vi "ManualMode.vi"(8 "error in (no error)":errorcluster, 10 "MainUI":refnum<queue>, 11 "ManualModeQueue":refnum<queue>) -> (0 "error out":errorcluster)   [LabVIEW 2019, in "ManualMode.lvlib"]
uses:
  ManualMode.lvlib
  Cluster - ManualModeMessageCluster.ctl
  Enum - ManualModeMessage.ctl
  MainController/Cluster - MainControllerMessage.ctl
  MainController/Enum - MainState.ctl
  Cluster - ManualModeData.ctl
  MainController/Cluster - HardwareConfiguration.ctl
  Cluster - ManualModeMonitorMessage.ctl
  Enum - ManualModeMonitorState.ctl
  Cluster - UIRefs.ctl
  Mark10 API/WriteSpeed.vi
  Mark10 API/WriteCWTravelLimit.vi
  Mark10 API/WriteCCWTravelLimit.vi
  Mark10 API/WriteStopMove.vi
  Mark10 API/WriteResetPositionToZero.vi
  MainController/MainController.lvlib
  Mark10 API/Mark 10 TSTM-DC.lvlib
  Utilites/Utilities.lvlib
panel:
  out "Work":dbl format="%.2f"
  out "Torque":dbl format="%.2f N"
  out "Position":dbl format="%.2f °"
  in  "GotoZero":bool
  in  "StopMove":bool
  in  "MoveCW":bool
  in  "MoveCCW":bool
  in  "SetZero":bool
  in  "Speed":dbl format="%.2f °/s"
  in  "Angle":dbl format="%.2f °"
  in  "CommandBar":cluster{"Start":bool, "Stop":bool}
  out "Wf":waveform(dbl)[](graph)
  in  "Pause":bool
  # "Mark 10 Control"
  # "Moves CW to 0"
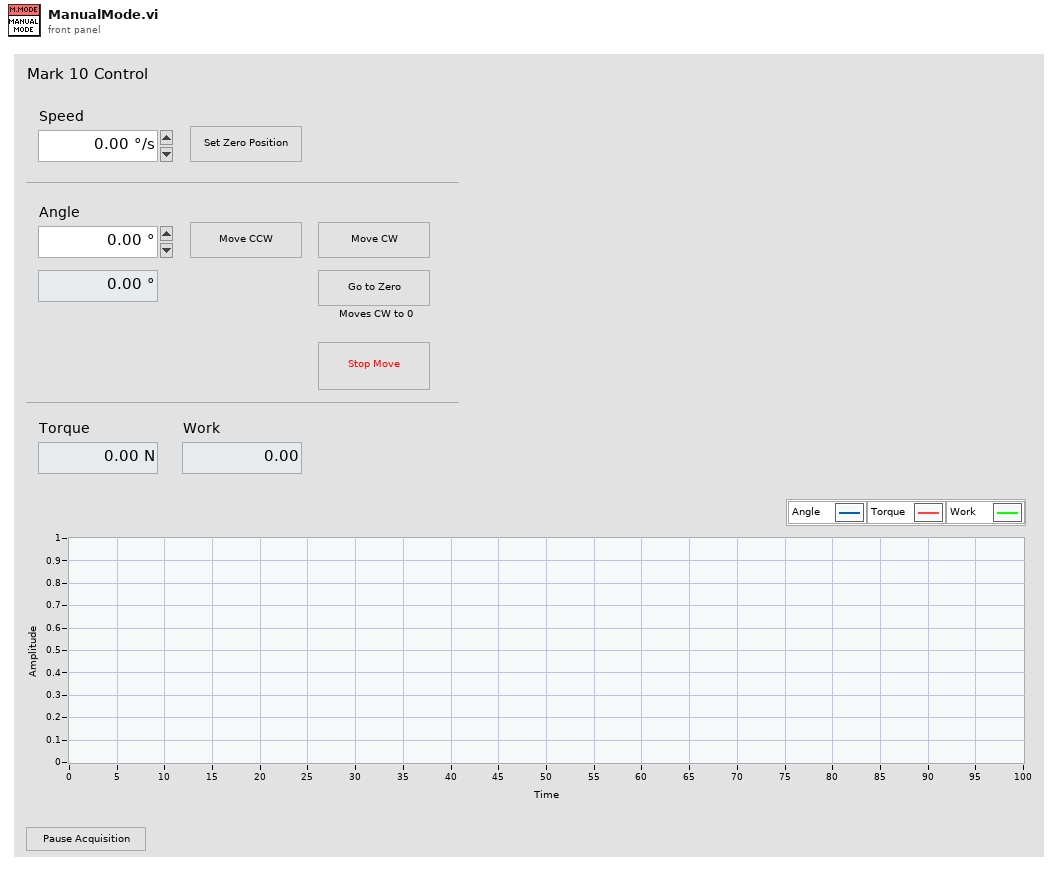
[diagram p1: front panel]
types:
  T1 = typedef "ManualMode.lvlib/Enum - ManualModeMonitorState.ctl" = enum16{"Idle", "SetCOM", "SetUIRefs", "Start", "Read", "Stop", "Pause", "Exit"}
  T2 = typedef "ManualMode.lvlib/Cluster - ManualModeMonitorMessage.ctl" = cluster{"Message":T1, "Data":variant}
  T3 = typedef "ManualMode.lvlib/Cluster - ManualModeData.ctl" = cluster{"Hardware Configuration":T4, "UIRefs":cluster{"Speed":refnum<vi>, "Angle":refnum<vi>}}
  T4 = typedef "MainController.lvlib/Cluster - HardwareConfiguration.ctl" = cluster{"Mark10COM":refnum<visa-resource-name>, "IsConnected":bool}
  T5 = typedef "ManualMode.lvlib/Enum - ManualModeMessage.ctl" = enum16{"Initialize", "Idle", "Start", "Stop", "Pause", "Resume", "BroadcastPreCollection", "MoveCCW", "MoveCW", "StopMove", "SetZero", "GotoZero", "UpdateHW", "Error", "Exit"}
  T6 = typedef "ManualMode.lvlib/Cluster - UIRefs.ctl" = cluster{"Work":refnum<vi>, "Torque":refnum<vi>, "Position":refnum<vi>, "Wf":refnum<vi>}
  T7 = typedef "MainController.lvlib/Enum - MainState.ctl" = enum16{"Initialize", "InitUIRefs", "LaunchSettings", "LaunchAutoMode", "LaunchManualMode", "LaunchTestReport", "ConnectHardware", "DisconnectHardware", "HiliteNavItems", "StartAutoMode", "PauseAutoMode", "StopAutoMode", "ShowFlyout", "HideFlyout", "BroadcastSettings", "PickupTestSettings", "BroadcastHW", "AutoTestDone", "DAQStatus", "UpdateCommandBar", "Error", "RecieveError", "Exit"}
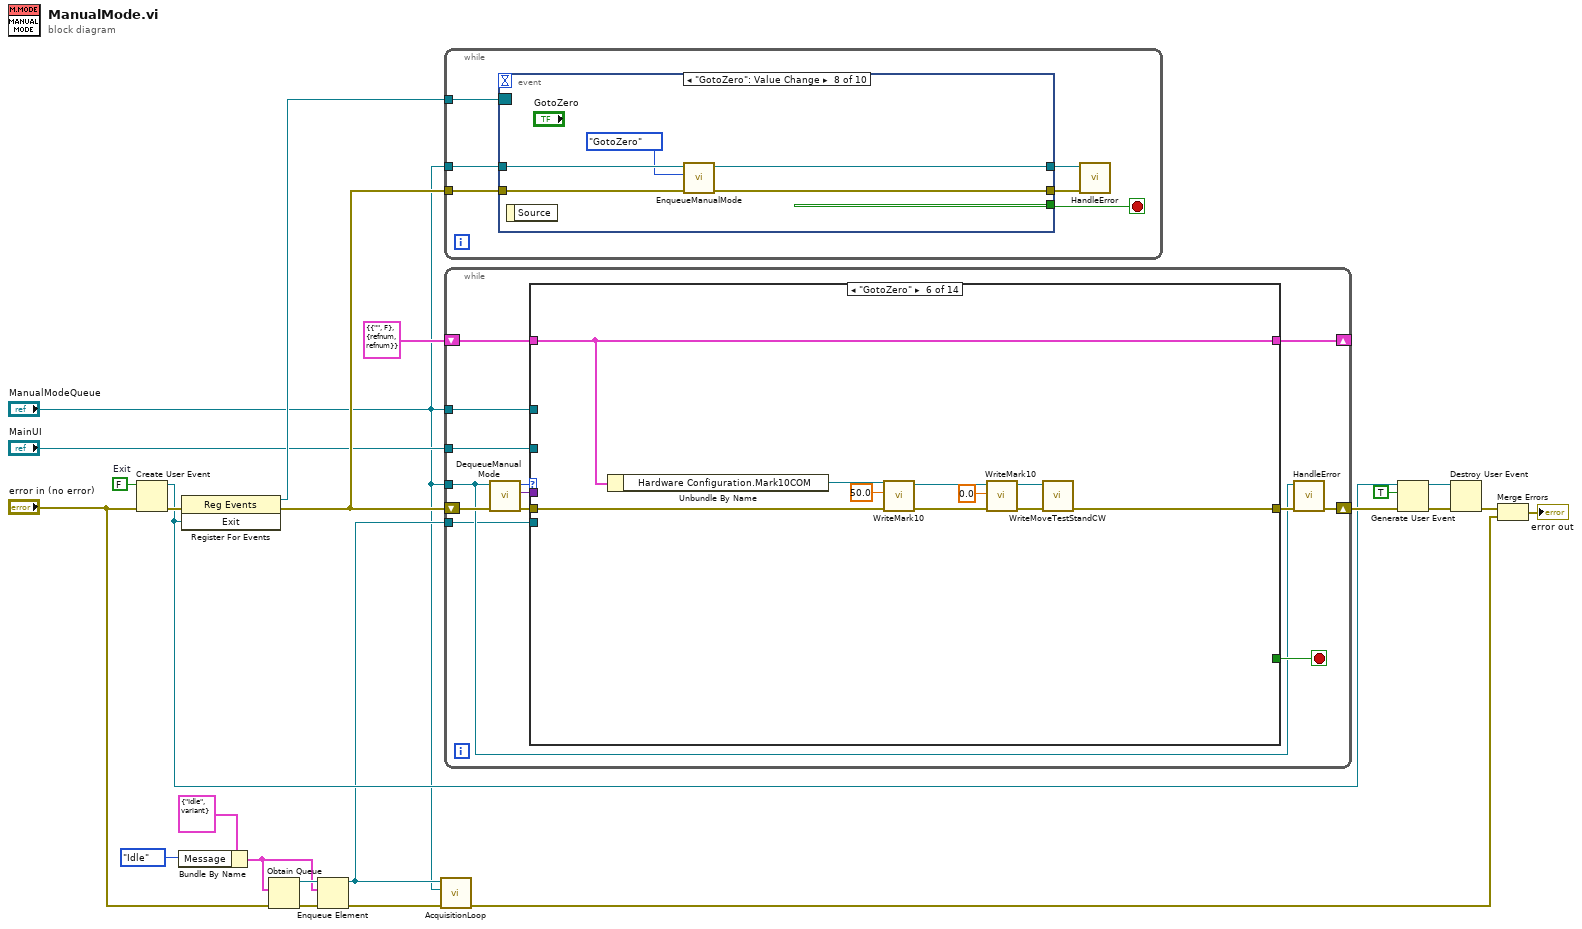
[diagram p0: block diagram]
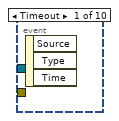
[diagram p2: hidden frame]
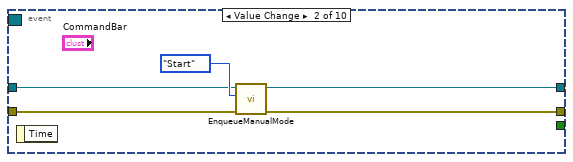
[diagram p3: hidden frame]
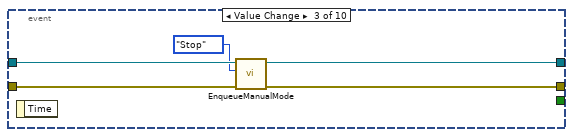
[diagram p4: hidden frame]
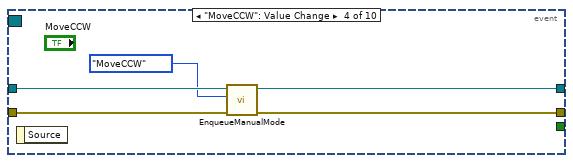
[diagram p5: hidden frame]
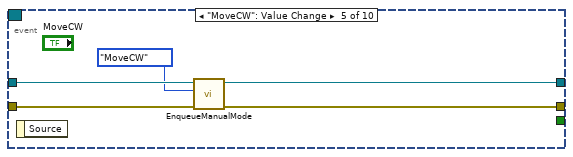
[diagram p6: hidden frame]
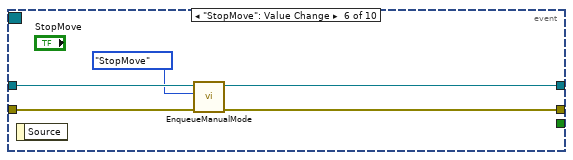
[diagram p7: hidden frame]
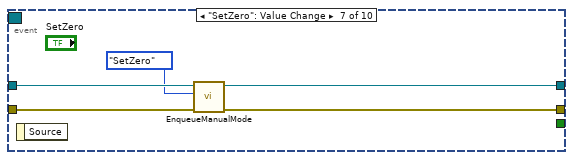
[diagram p8: hidden frame]
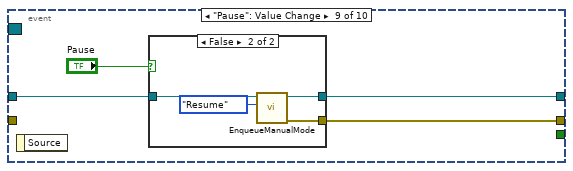
[diagram p9: hidden frame]
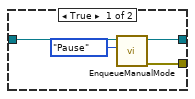
[diagram p10: hidden frame]
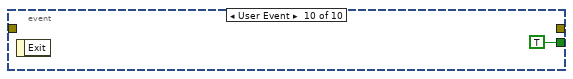
[diagram p11: hidden frame]
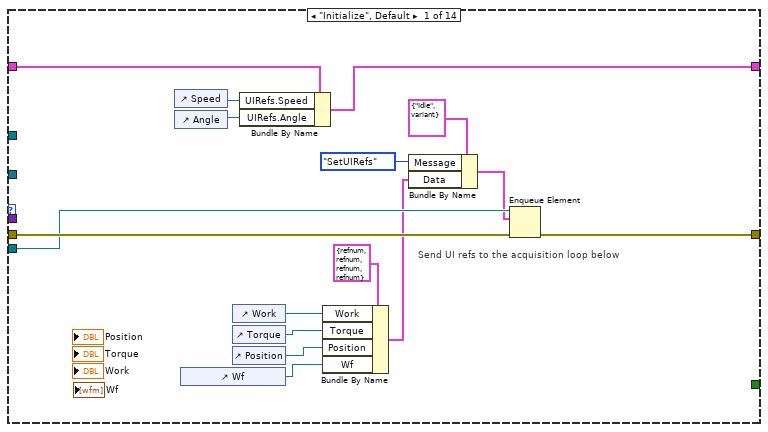
[diagram p12: hidden frame]
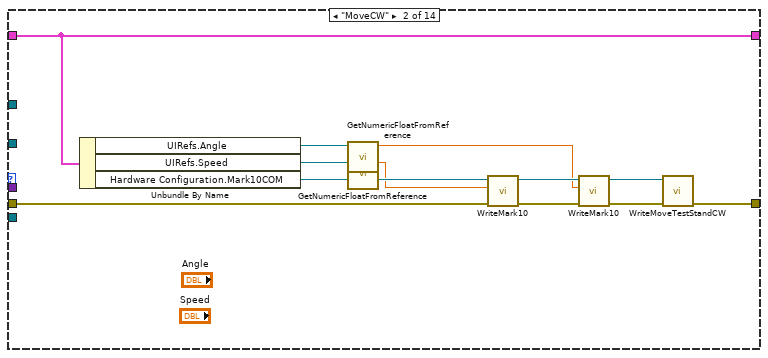
[diagram p13: hidden frame]
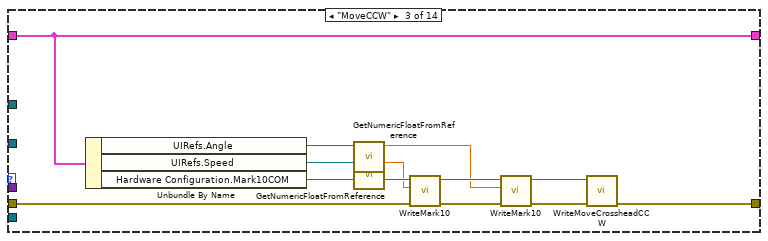
[diagram p14: hidden frame]
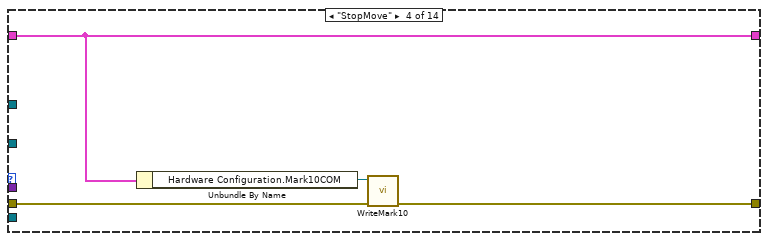
[diagram p15: hidden frame]
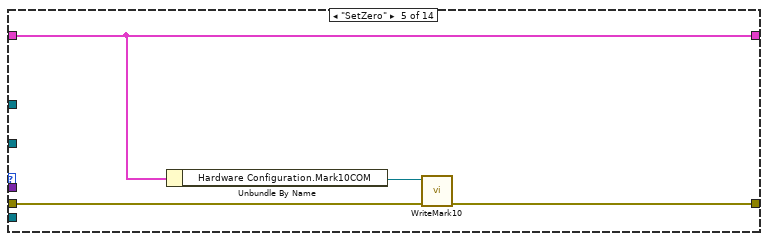
[diagram p16: hidden frame]
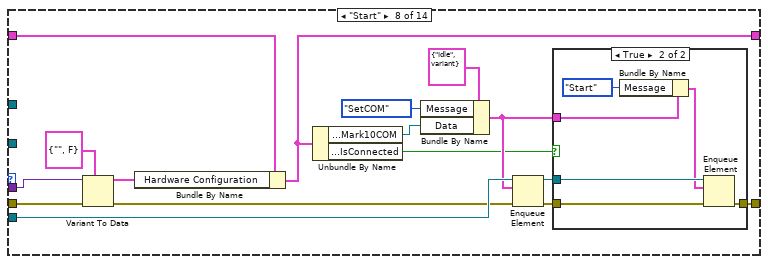
[diagram p18: hidden frame]
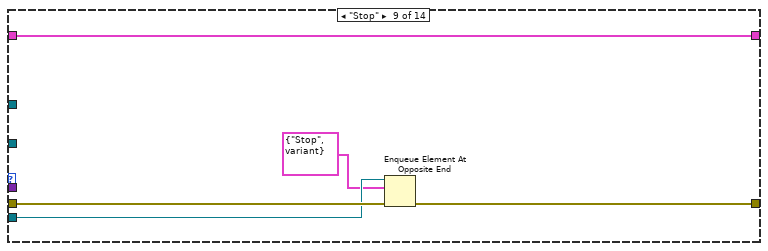
[diagram p20: hidden frame]
diagram:
  w22 = FALSE  # Exit
  n1 = Create User Event(user event datatype=w22, error in="error in (no error)") -> (user event=w19:refnum<user-event>, error out=w23:errorcluster)
  n2 = Bundle By Name(cluster=T2 {"Message"=enum."Idle", "Data"=variant}, "Message"=Enum_-_ManualModeMonitorState."Idle") -> (w6:T2)
  n3 = register-events(error in=w23, w19) -> (reference out=w21:refnum<event-registration>, error out=w14:errorcluster)  [unwired: 1 in]
  n4 = Obtain Queue(element data type=w6, error in (no error)="error in (no error)") -> (queue out=w10:refnum<queue>, error out=w11:errorcluster)  [unwired: 3 in, 1 out]
  n5 = Enqueue Element(queue=w10, element=w6, error in (no error)=w11) -> (queue out=w5:refnum<queue>, error out=w9:errorcluster)  [unwired: 1 in, 1 out]
  n6 = call "AcquisitionLoop.vi"("error in (no error)"=w9, "ManualModeQueue"="ManualModeQueue", "AcquisitionQueue"=w5) -> ("Error Out"=w3:errorcluster)  [unwired: 8 in]
  n7 = while {
    tunnel: w21 -> [w29]
    tunnel: w14 -> [w27]
    tunnel: "ManualModeQueue" -> [w26]
    stop <- w28 stop-if-true
    n8 = event shown="[7] \"GotoZero\": Value Change" {
      selector: w29 -> [_ _ _ _ _ _ _ _ _ _]
      dyn-events: _ -> [_ _ _ _ _ _ _ _ _ _]
      timeout: _ -> [_ _ _ _ _ _ _ _ _ _]
      tunnel: [_ _ _ _ _ _ _ _ _ TRUE] -> w28
      tunnel: w27 -> [_ w34 w39 w43 w48 w53 w58 w63 _ _]
      tunnel: w26 -> [_ w32 w38 w44 w49 w54 w59 w64 w68 _]
      tunnel: [_ w30 w35 w40 w45 w50 w55 w60 w67 _] -> w25
      tunnel: [_ w31 w36 w41 w46 w51 w56 w61 w66 _] -> w24
      event Timeout {
        n9 = event-data() -> ()  [unwired: 1 in, 3 out]
      }
      event "CommandBar.Start": Value Change {
        n10 = event-data() -> ()  [unwired: 1 in, 1 out]
        n11 = call "EnqueueManualMode.vi"("error in (no error)"=w34, "Message"=Enum_-_ManualModeMessage."Start" ("PreCollectionMessage"), "queue"=w32) -> ("error out"=w30:errorcluster, "queue out"=w31:refnum<queue>)  [unwired: 7 in]
      }
      event "CommandBar.Stop": Value Change {
        n12 = event-data() -> ()  [unwired: 1 in, 1 out]
        n13 = call "EnqueueManualMode.vi"("error in (no error)"=w39, "Message"=Enum_-_ManualModeMessage."Stop" ("PreCollectionMessage"), "queue"=w38) -> ("error out"=w35:errorcluster, "queue out"=w36:refnum<queue>)  [unwired: 7 in]
      }
      event "MoveCCW": Value Change {
        n14 = event-data() -> ()  [unwired: 1 in, 1 out]
        n15 = call "EnqueueManualMode.vi"("error in (no error)"=w43, "Message"=Enum_-_ManualModeMessage."MoveCCW", "queue"=w44) -> ("error out"=w40:errorcluster, "queue out"=w41:refnum<queue>)  [unwired: 7 in]
      }
      event "MoveCW": Value Change {
        n16 = event-data() -> ()  [unwired: 1 in, 1 out]
        n17 = call "EnqueueManualMode.vi"("error in (no error)"=w48, "Message"=Enum_-_ManualModeMessage."MoveCW", "queue"=w49) -> ("error out"=w45:errorcluster, "queue out"=w46:refnum<queue>)  [unwired: 7 in]
      }
      event "StopMove": Value Change {
        n18 = event-data() -> ()  [unwired: 1 in, 1 out]
        n19 = call "EnqueueManualMode.vi"("error in (no error)"=w53, "Message"=Enum_-_ManualModeMessage."StopMove", "queue"=w54) -> ("error out"=w50:errorcluster, "queue out"=w51:refnum<queue>)  [unwired: 7 in]
      }
      event "SetZero": Value Change {
        n20 = event-data() -> ()  [unwired: 1 in, 1 out]
        n21 = call "EnqueueManualMode.vi"("error in (no error)"=w58, "Message"=Enum_-_ManualModeMessage."SetZero", "queue"=w59) -> ("error out"=w55:errorcluster, "queue out"=w56:refnum<queue>)  [unwired: 7 in]
      }
      event "GotoZero": Value Change {
        n22 = event-data() -> ()  [unwired: 1 in, 1 out]
        n23 = call "EnqueueManualMode.vi"("error in (no error)"=w63, "Message"=Enum_-_ManualModeMessage."GotoZero", "queue"=w64) -> ("error out"=w60:errorcluster, "queue out"=w61:refnum<queue>)  [unwired: 7 in]
      }
      event "Pause": Value Change {
        n24 = event-data() -> ()  [unwired: 1 in, 1 out]
        n25 = case shown="False" "Pause" {
          tunnel: w68 -> [w72 w76]
          tunnel: [w70 w74] -> w67
          tunnel: [w69 w73] -> w66
          frame True {
            n26 = call "EnqueueManualMode.vi"("Message"=Enum_-_ManualModeMessage."Pause", "queue"=w72) -> ("error out"=w70:errorcluster, "queue out"=w69:refnum<queue>)  [unwired: 8 in]
          }
          frame False {
            n27 = call "EnqueueManualMode.vi"("Message"=Enum_-_ManualModeMessage."Resume", "queue"=w76) -> ("error out"=w74:errorcluster, "queue out"=w73:refnum<queue>)  [unwired: 8 in]
          }
        }
      }
      event User Event {
        n28 = event-data() -> ()  [unwired: 1 in, 1 out]
      }
    }
    n29 = call "HandleError.vi"("error in (no error)"=w25, "queue"=w24) -> ()  [unwired: 8 in, 2 out]
  }
  n30 = while {
    tunnel: "ManualModeQueue" -> [w79]
    shift-right: [w80] -> w20
    shift-left: w14 -> [w90]
    shift-right: [w85] -> _
    shift-left: T3 {"Hardware Configuration"={"Mark10COM"="", "IsConnected"=FALSE}, "UIRefs"={"Speed"=refnum, "Angle"=refnum}} -> [w86]
    tunnel: "MainUI" -> [w83]
    tunnel: "ManualModeQueue" -> [w82]
    tunnel: w5 -> [w78]
    stop <- w87 stop-if-true
    n31 = call "DequeueManualMode.vi"("error in (no error)"=w90, "Queue in"=w79) -> ("error out"=w88:errorcluster, "Data"=w89:variant, "State"=w84:T5)  [unwired: 7 in]
    n32 = case shown="\"GotoZero\"" w84 {
      tunnel: w89 -> [_ _ _ _ _ _ _ w158 _ _ _ w198 w203 _]
      tunnel: [w105 w112 w126 w133 w137 w140 w150 w162 w176 w181 w186 w194 w207 w212] -> w81
      tunnel: w88 -> [w106 w116 w130 w134 w138 w145 w150 w166 w177 w183 w188 w200 w202 _]
      tunnel: [_ _ _ _ _ _ _ _ _ _ _ _ _ TRUE] -> w87
      tunnel: w86 -> [w93 w118 w122 w132 w136 w147 w149 w153 w178 w182 w187 w195 w208 w213]
      tunnel: [w94 w118 w122 w132 w136 w147 w149 w154 w178 w182 w187 w196 w208 w213] -> w85
      tunnel: w83 -> [_ _ _ _ _ _ _ _ _ _ _ _ w206 _]
      tunnel: w82 -> [_ _ _ _ _ _ _ _ _ _ _ _ _ _]
      tunnel: w78 -> [w104 _ _ _ _ _ _ w165 w175 w180 w185 w193 _ w211]
      frame "Initialize", Default {
        # "Send UI refs to the acquisition loop below"
        n33 = control-ref of="Speed"() -> (w92:refnum<vi>)
        n34 = control-ref of="Angle"() -> (w91:refnum<vi>)
        n35 = control-ref of="Wf"() -> (w103:refnum<vi>)
        n36 = control-ref of="Work"() -> (w100:refnum<vi>)
        n37 = control-ref of="Torque"() -> (w101:refnum<vi>)
        n38 = control-ref of="Position"() -> (w102:refnum<vi>)
        n39 = Bundle By Name(cluster=w93, "UIRefs.Speed"=w92, "UIRefs.Angle"=w91) -> (w94:T3)
        n40 = Bundle By Name(cluster=T6 {"Work"=refnum, "Torque"=refnum, "Position"=refnum, "Wf"=refnum} ("output cluster"), "Work"=w100, "Torque"=w101, "Position"=w102, "Wf"=w103) -> (w95:T6)
        n41 = Bundle By Name(cluster=T2 {"Message"=enum."Idle", "Data"=variant}, "Message"=Enum_-_ManualModeMonitorState."SetUIRefs", "Data"=w95) -> (w97:T2)
        n42 = Enqueue Element(queue=w104, element=w97, error in (no error)=w106) -> (error out=w105:errorcluster)  [unwired: 1 in, 2 out]
      }
      frame "MoveCW" {
        n43 = Unbundle By Name(w118) -> ("UIRefs.Angle"=w110:refnum<vi>, "UIRefs.Speed"=w108:refnum<vi>, "Hardware Configuration.Mark10COM"=w117:refnum<visa-resource-name>)
        n44 = call "GetNumericFloatFromReference.vi"("reference"=w110) -> ("Value"=w109:dbl)  [unwired: 9 in, 1 out]
        n45 = call "GetNumericFloatFromReference.vi"("reference"=w108) -> ("Value"=w107:dbl)  [unwired: 9 in, 1 out]
        n46 = call-poly "WriteMark10.vi"("error in"=w116, "Speed"=w107, "VISA resource name"=w117) -> ("error out"=w115:errorcluster, "VISA resource name out"=w114:refnum<visa-resource-name>)  [unwired: 7 in]
        n47 = call-poly "WriteMark10.vi"("error in"=w115, "CWTravelLimit"=w109, "VISA resource name"=w114) -> ("error out"=w113:errorcluster, "VISA resource name out"=w111:refnum<visa-resource-name>)  [unwired: 7 in]
        n48 = call "WriteMoveTestStandCW.vi"("error in"=w113, "VISA resource name"=w111) -> ("error out"=w112:errorcluster)  [unwired: 8 in, 1 out]
      }
      frame "MoveCCW" {
        n49 = Unbundle By Name(w122) -> ("UIRefs.Angle"=w124:refnum<vi>, "UIRefs.Speed"=w123:refnum<vi>, "Hardware Configuration.Mark10COM"=w121:refnum<visa-resource-name>)
        n50 = call "GetNumericFloatFromReference.vi"("reference"=w124) -> ("Value"=w119:dbl)  [unwired: 9 in, 1 out]
        n51 = call "GetNumericFloatFromReference.vi"("reference"=w123) -> ("Value"=w120:dbl)  [unwired: 9 in, 1 out]
        n52 = call-poly "WriteMark10.vi"("error in"=w130, "Speed"=w120, "VISA resource name"=w121) -> ("error out"=w129:errorcluster, "VISA resource name out"=w128:refnum<visa-resource-name>)  [unwired: 7 in]
        n53 = call-poly "WriteMark10.vi"("error in"=w129, "CCWTravelLimit"=w119, "VISA resource name"=w128) -> ("error out"=w127:errorcluster, "VISA resource name out"=w125:refnum<visa-resource-name>)  [unwired: 7 in]
        n54 = call "WriteMoveCrossheadCCW.vi"("error in"=w127, "VISA resource name"=w125) -> ("error out"=w126:errorcluster)  [unwired: 8 in, 1 out]
      }
      frame "StopMove" {
        n55 = Unbundle By Name(w132) -> ("Hardware Configuration.Mark10COM"=w131:refnum<visa-resource-name>)
        n56 = call-poly "WriteMark10.vi"("error in"=w134, "VISA resource name"=w131) -> ("error out"=w133:errorcluster)  [unwired: 8 in, 1 out]
      }
      frame "SetZero" {
        n57 = Unbundle By Name(w136) -> ("Hardware Configuration.Mark10COM"=w135:refnum<visa-resource-name>)
        n58 = call-poly "WriteMark10.vi"("error in"=w138, "VISA resource name"=w135) -> ("error out"=w137:errorcluster)  [unwired: 8 in, 1 out]
      }
      frame "GotoZero" {
        n59 = Unbundle By Name(w147) -> ("Hardware Configuration.Mark10COM"=w144:refnum<visa-resource-name>)
        n60 = call-poly "WriteMark10.vi"("error in"=w145, "Speed"=50.0, "VISA resource name"=w144) -> ("error out"=w142:errorcluster, "VISA resource name out"=w143:refnum<visa-resource-name>)  [unwired: 7 in]
        n61 = call-poly "WriteMark10.vi"("error in"=w142, "CWTravelLimit"=0.0, "VISA resource name"=w143) -> ("error out"=w148:errorcluster, "VISA resource name out"=w139:refnum<visa-resource-name>)  [unwired: 7 in]
        n62 = call "WriteMoveTestStandCW.vi"("error in"=w148, "VISA resource name"=w139) -> ("error out"=w140:errorcluster)  [unwired: 8 in, 1 out]
      }
      frame "Idle" {
      }
      frame "Start" {
        n63 = Variant To Data(error in=w166, type=T4 {"Mark10COM"="", "IsConnected"=FALSE} ("Hardware Configuration"), Variant=w158) -> (data=w155:T4, error out=w156:errorcluster)
        n64 = Bundle By Name(cluster=w153, "Hardware Configuration"=w155) -> (w154:T3)
        n65 = Unbundle By Name(w154) -> ("Hardware Configuration.Mark10COM"=w159:refnum<visa-resource-name>, "Hardware Configuration.IsConnected"=w151:bool)
        n66 = Bundle By Name(cluster=T2 {"Message"=enum."Idle", "Data"=variant}, "Message"=Enum_-_ManualModeMonitorState."SetCOM", "Data"=w159) -> (w152:T2)
        n67 = Enqueue Element(queue=w165, element=w152, error in (no error)=w156) -> (queue out=w164:refnum<queue>, error out=w163:errorcluster)  [unwired: 1 in, 1 out]
        n68 = case shown="True" w151 {
          tunnel: w164 -> [_ w173]
          tunnel: w163 -> [w167 w172]
          tunnel: [w167 w171] -> w162
          tunnel: w152 -> [_ w168]
          frame False {
          }
          frame True {
            n69 = Bundle By Name(cluster=w168, "Message"=Enum_-_ManualModeMonitorState."Start") -> (w169:T2)
            n70 = Enqueue Element(queue=w173, element=w169, error in (no error)=w172) -> (error out=w171:errorcluster)  [unwired: 1 in, 2 out]
          }
        }
      }
      frame "Stop" {
        n71 = Enqueue Element At Opposite End(queue=w175, element=T2 {"Message"=enum."Stop", "Data"=variant}, error in (no error)=w177) -> (error out=w176:errorcluster)  [unwired: 1 in, 2 out]
      }
      frame "Pause" {
        n72 = Enqueue Element(queue=w180, element=T2 {"Message"=enum."Pause", "Data"=variant}, error in (no error)=w183) -> (error out=w181:errorcluster)  [unwired: 1 in, 2 out]
      }
      frame "Resume" {
        n73 = Enqueue Element(queue=w185, element=T2 {"Message"=enum."Start", "Data"=variant}, error in (no error)=w188) -> (error out=w186:errorcluster)  [unwired: 1 in, 2 out]
      }
      frame "UpdateHW" {
        n74 = Variant To Data(error in=w200, type=T4 {"Mark10COM"="", "IsConnected"=FALSE} ("Hardware Configuration"), Variant=w198) -> (data=w192:T4, error out=w199:errorcluster)
        n75 = Unbundle By Name(w192) -> ("Mark10COM"=w191:refnum<visa-resource-name>)
        n76 = Bundle By Name(cluster=w195, "Hardware Configuration"=w192) -> (w196:T3)
        n77 = Bundle By Name(cluster=T2 {"Message"=enum."SetCOM", "Data"=variant} ("element"), "Data"=w191) -> (w189:T2)
        n78 = Enqueue Element(queue=w193, element=w189, error in (no error)=w199) -> (error out=w194:errorcluster)  [unwired: 1 in, 2 out]
      }
      frame "Error" {
        # "Forward error to main controller"
        n79 = Variant To Data(error in=w202, type=w202, Variant=w203) -> (data=w201:errorcluster, error out=w204:errorcluster)
        n80 = call "EnqueueMainController.vi"("error in (no error)"=w204, "Data"=w201, "Message"=Enum_-_MainState."RecieveError", "MainQueue"=w206) -> ("error out"=w207:errorcluster)  [unwired: 5 in, 2 out]
      }
      frame "Exit" {
        n81 = Lossy Enqueue Element(queue=w211, element=T2 {"Message"=enum."Exit", "Data"=variant}, error in (no error)=errorcluster {"status"=FALSE, "code"=0, "source"=""}) -> (error out=w212:errorcluster)  [unwired: 3 out]
      }
    }
    n82 = call "HandleError.vi"("error in (no error)"=w81, "queue"=w79) -> ("error out"=w80:errorcluster)  [unwired: 8 in, 1 out]
  }
  n83 = Generate User Event(user event=w19, event data cluster=TRUE ("event data"), error in=w20) -> (user event out=w17:refnum<user-event>, error out=w18:errorcluster)  [unwired: 1 in]
  n84 = Destroy User Event(user event=w17, error in=w18) -> (error out=w4:errorcluster)
  n85 = Merge Errors(w4, w3) -> (→"error out":errorcluster)
